vi "FlatToRichnixnet_grpc_BlinkRequest.vi"(5 "OutputClusterType":T1, 11 "InputCluster":T3) -> (3 "OutputCluster":T1)   [LabVIEW 2025, in "xnet-grpc_client.lvlib"]
uses:
  nixnet_grpc_BlinkRequest_Flat.ctl
  nidevice_grpc_Session_Flat.ctl
  nixnet_grpc_BlinkMode.ctl
  nixnet_grpc_BlinkRequest.ctl
  nixnet_grpc_BlinkRequest_modifier_enum/nixnet_grpc_BlinkRequest_modifier_enum.lvclass
  nidevice_grpc_Session.ctl
  xnet-grpc_client.lvlib
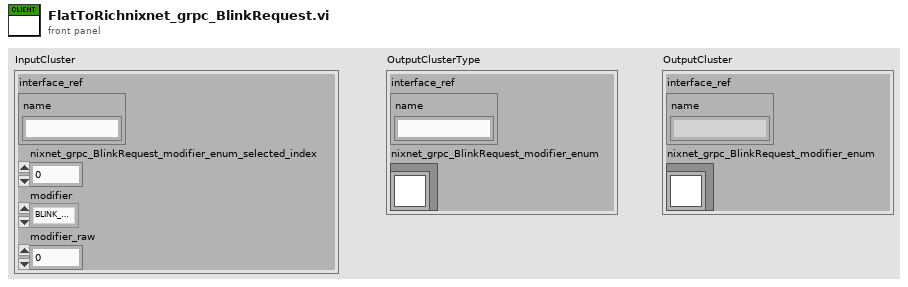
[diagram p1: front panel]
types:
  T1 = typedef "xnet-grpc_client.lvlib/nixnet_grpc_BlinkRequest.ctl" = cluster{"interface_ref":T2, "nixnet_grpc_BlinkRequest_modifier_enum":refnum<class "nixnet_grpc_BlinkRequest_modifier_enum.lvclass">}
  T2 = typedef "xnet-grpc_client.lvlib/nidevice_grpc_Session.ctl" = cluster{"name":string}
  T3 = typedef "xnet-grpc_client.lvlib/nixnet_grpc_BlinkRequest_Flat.ctl" = cluster{"interface_ref":T4, "nixnet_grpc_BlinkRequest_modifier_enum_selected_index":i32, "modifier":T5, "modifier_raw":u32}
  T4 = typedef "xnet-grpc_client.lvlib/nidevice_grpc_Session_Flat.ctl" = cluster{"name":string}
  T5 = typedef "xnet-grpc_client.lvlib/nixnet_grpc_BlinkMode.ctl" = enum32{"BLINK_MODE_DISABLE", "BLINK_MODE_ENABLE"}
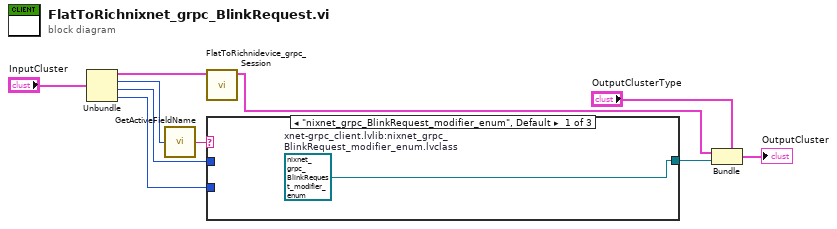
[diagram p0: block diagram]
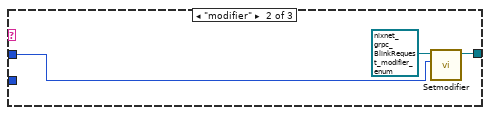
[diagram p2: hidden frame]
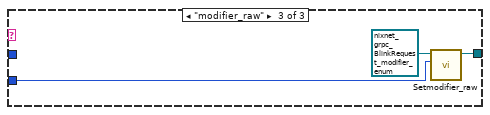
[diagram p3: hidden frame]
diagram:
  n1 = Unbundle "Unbundle"("InputCluster") -> ("interface_ref"=w7:T4, "nixnet_grpc_BlinkRequest_modifier_enum_selected_index"=w5:i32, "modifier"=w2:T5, "modifier_raw"=w1:u32)
  n2 = call "GetActiveFieldName.vi"("protobuf index"=w5) -> ("oneof field name"=w4:string)
  n3 = call "FlatToRichnidevice_grpc_Session.vi"("InputCluster"=w7) -> ("OutputCluster"=w6:T2)  [unwired: 10 in]
  n4 = case "nixnet_grpc_BlinkRequest_modifier_enum" shown="\"nixnet_grpc_BlinkRequest_modifier_enum\", Default" w4 {
    tunnel: [w11 w13 w16] -> w3
    tunnel: w2 -> [_ w14 _]
    tunnel: w1 -> [_ _ w17]
    frame "nixnet_grpc_BlinkRequest_modifier_enum", Default {
      w11 = refnum<class "nixnet_grpc_BlinkRequest_modifier_enum.lvclass"> refnum  # xnet-grpc_client.lvlib:nixnet_grpc_BlinkRequest_modifier_enum.lvclass
    }
    frame "modifier" {
      n5 = call "Setmodifier.vi"("Set_Val"=w14, "OneOfTemplate in"=refnum<class "nixnet_grpc_BlinkRequest_modifier_enum.lvclass"> refnum) -> ("OneOfTemplate out"=w13:refnum<class "nixnet_grpc_BlinkRequest_modifier_enum.lvclass">)  [unwired: 8 in, 1 out]
    }
    frame "modifier_raw" {
      n6 = call "Setmodifier_raw.vi"("Set_Val"=w17, "OneOfTemplate in"=refnum<class "nixnet_grpc_BlinkRequest_modifier_enum.lvclass"> refnum) -> ("OneOfTemplate out"=w16:refnum<class "nixnet_grpc_BlinkRequest_modifier_enum.lvclass">)  [unwired: 8 in, 1 out]
    }
  }
  n7 = Bundle "Bundle"(cluster="OutputClusterType", "interface_ref"=w6, "nixnet_grpc_BlinkRequest_modifier_enum"=w3) -> (→"OutputCluster":T1)
